vi "WaitMinTimeBetweenCalls_1.vi"(2 "Minimum ms between calls":i32=5000) -> ()   [LabVIEW 2012, in "MyHostCode.lvlib"]
doc: "This VI ensures a minimum amount of time has passed between calls. If the minimum amount of time has not passed when this VI is called, this VI waits the remaining amount of time. If more then the minimum time has passed, this VI returns immeadiately without yielding the processor."
uses:
  MyHostCode.lvlib
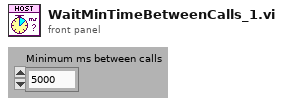
[diagram p1: front panel]
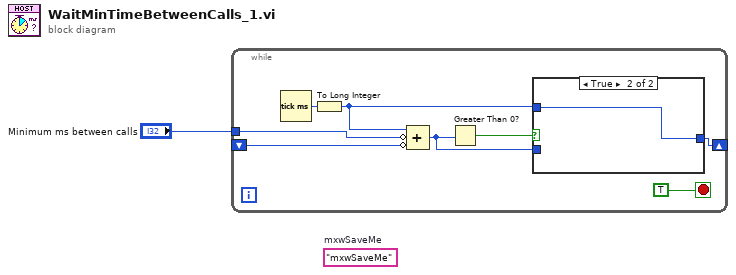
[diagram p0: block diagram]
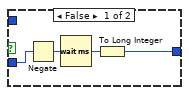
[diagram p2: hidden frame]
diagram:
  (unwired) "mxwSaveMe"  # mxwSaveMe
  n1 = while {
    shift-right: [w7] -> _
    shift-left: _ -> [w2]
    tunnel: "Minimum ms between calls" -> [w3]
    stop <- TRUE stop-if-true
    n2 = Tick Count (ms)() -> (millisecond timer value=w9:u32)
    n3 = To Long Integer(number=w9) -> (32bit integer=w6:i32)
    n4 = Compound Arithmetic op=ADD(w6, invert w3, invert w2) -> (w5:i32)
    n5 = Greater Than 0?(x=w5) -> (x > 0?=w4:bool)
    n6 = case shown="True" w4 {
      tunnel: w5 -> [w13 _]
      tunnel: w6 -> [_ w14]
      tunnel: [w10 w14] -> w7
      frame False {
        n7 = Negate(x=w13) -> (-x=w12:i32)
        n8 = Wait (ms)(milliseconds to wait=w12) -> (millisecond timer value=w11:u32)
        n9 = To Long Integer(number=w11) -> (32bit integer=w10:i32)
      }
      frame True {
      }
    }
  }
